vi "Generate Error.vi"(0 "Error Code":i32, 11 "error in (no error)":errorcluster) -> (15 "error out":errorcluster)   [LabVIEW 2024]
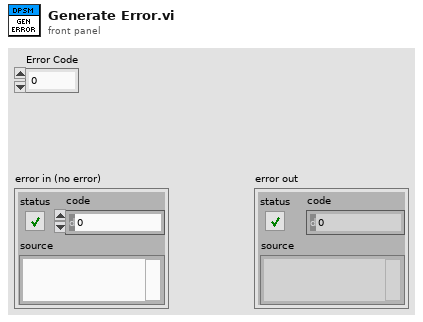
[diagram p1: front panel]
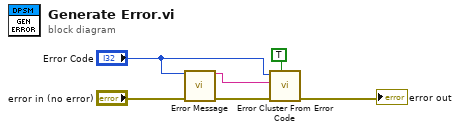
[diagram p0: block diagram]
diagram:
  n1 = call "Error Message.vi"("Error Code"="Error Code", "error in (no error)"="error in (no error)") -> ("Error Message"=w5:string, "error out"=w6:errorcluster)  [unwired: 11 in, 1 out]
  n2 = call <vilib>:"Error Cluster From Error Code.vi"("show call chain? (False)"=TRUE, "error in (no error)"=w6, "error message (\"\")"=w5, "error code (0)"="Error Code") -> ("error out"=→"error out":errorcluster)  [unwired: 5 in]
